vi "GetDnetA Input.vi"   [LabVIEW 2011]
uses:
  GlobalVariables.vi
  DS/DSRead uint16.vi
types:
  T1 = enum16{"OPC Server", "Global", "Dnet1", "Dnet2", "Dnet3", "Ain1", "Ain2", "Aout1", "Din1", "Din2", "Dout1"}
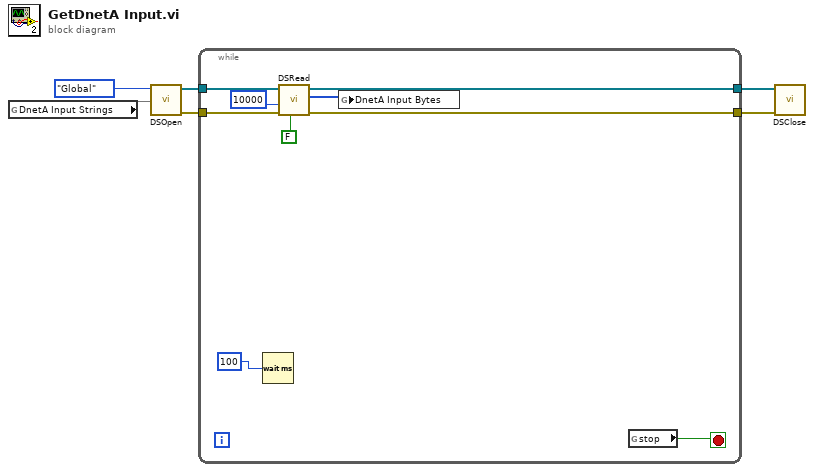
[diagram p0: block diagram]
diagram:
  n1 = global read "GlobalVariables.vi" "DnetA Input Strings"() -> (w5)
  n2 = call "DSOpen.vi"("Array"=w5, "Slot"=T1."Global") -> ("error Out"=w4:errorcluster[], "connection out"=w3:refnum<k13>[])  [unwired: 8 in]
  n3 = while {
    tunnel: w4 -> [w14]
    tunnel: w3 -> [w13]
    tunnel: [w10] -> w2
    tunnel: [w9] -> w1
    stop <- w15 stop-if-true
    n4 = Wait (ms)(milliseconds to wait=100) -> ()  [unwired: 1 out]
    n5 = call-poly "DSRead.vi"("wait for updated value (T)"=FALSE, "error in"=w14, "ms timeout (10000)"=10000, "connection in"=w13) -> ("error out"=w9:errorcluster[], "data"=w7:u16[], "connection out"=w10:refnum<k13>[])  [unwired: 5 in]
    n6 = global write "GlobalVariables.vi" "DnetA Input Bytes"(w7) -> ()
    n7 = global read "GlobalVariables.vi" "stop"() -> (w15:bool)
  }
  n8 = call "DSClose.vi"("error in (no error)"=w1, "connection id"=w2) -> ()  [unwired: 10 in]
